vi "ConfigureDlg.vi"(8 "error in (no error)":errorcluster, 11 "PXI_MultiTrig in":refnum<class "PXI_MultiTrig.lvclass">) -> (0 "error out":errorcluster, 2 "Changed?":bool, 3 "PXI_MultiTrig out":refnum<class "PXI_MultiTrig.lvclass">)   [LabVIEW 2018, in "SyncPlugins.lvlib" / "PXI_MultiTrig.lvclass"]
uses:
  PXI_MultiTrig.lvclass
  C:/Program Files/National Instruments/LabVIEW 2018/user.lib/NIST/BaseClasses/BasePlugin_class/BasePlugin.lvclass
  Typedefs/clClocks.ctl
  Typedefs/clTrigger.ctl
  Typedefs/TimeRefType.ctl
  PXI_MultiTrig.lvclass/PXI_MultiTrig.ctl
  <userlib>/NIST/BaseClasses/BasePlugin_class/BasePlugin.lvclass/BasePlugin.ctl
  Accessors/Read RefClkHandle.vi
  Accessors/Read TimingHandle.vi
  Accessors/Read Clocks.vi
  Accessors/Read Triggers.vi
  Accessors/Read TimeRefType.vi
  Accessors/Read SyncWindowsClock.vi
  Accessors/Read RefClkSource.vi
  Accessors/Write RefClkHandle.vi
  Accessors/Write TimingHandle.vi
  Accessors/Write Clocks.vi
  Accessors/Write Triggers.vi
  <userlib>/NIST/BaseClasses/BasePlugin_class/Accessors/Read PluginIniFilePath.vi
  Accessors/Write TimeRefType.vi
  Accessors/Write SyncWindowsClock.vi
  Accessors/Write RefClkSource.vi
  <userlib>/NIST/BaseClasses/BasePlugin_class/Accessors/Write PluginIniFilePath.vi
  <vilib>/Utility/config.llb/NI_LVConfig.lvlib
panel:
  in  "btnSaveAs":bool
  in  "btnSave":bool
  in  "Tab Control":T1(tab)
  in  "TimingCard":string="PXI1Slot7"
  in  "TimeRefType":T2=enum."GPS"
  in  "SyncWinClk":bool caption="Synchronize Windows Clock"
  in  "RefClkSource":string="PXI_Trig0"
  in  "RefClkCard":string="PXI1Slot7"
  in  "Clocks":T3[](array[typedef])
  in  "Triggers":T4[](array[typedef]) {"Invert?" items=["Don't Invert Signal", "Invert Signal"]; "Edge" items=["Rising Edge", "Falling Edge"]}
  in  "btnCancel":bool
  # "Windows clock synchronization\nrequires LabVIEW to be running\nas Administrator"
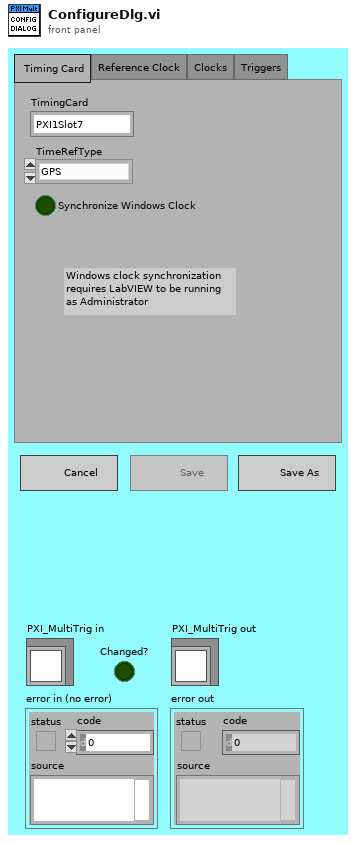
[diagram p1: front panel]
types:
  T1 = enum32{" Timing Card", "Reference Clock", "Clocks", "Triggers"}
  T2 = typedef "SyncPlugins.lvlib/PXI_MultiTrig.lvclass/TimeRefType.ctl" = enum16{"1588", "Free Running", "GPS", "IRIG", "PPS"}
  T3 = typedef "SyncPlugins.lvlib/PXI_MultiTrig.lvclass/clClocks.ctl" = cluster{"Name":string, "RefClk":string, "ClkTerminal":string, "Frequency":dbl, "DutyCycle":dbl, "ClkType":string, "Initiated":bool, "TrigTime":bool}
  T4 = typedef "SyncPlugins.lvlib/PXI_MultiTrig.lvclass/clTrigger.ctl" = cluster{"Name":string, "DestTerm":string, "SrcTerm":string, "SyncClk":string, "Edge":i32, "Invert?":i32, "Initiated":bool, "Type":string, "TrigTime":bool}
  T5 = enum8{"Enabled", "Disabled", "Disabled and Grayed Out"}
  T6 = enum32{"Invalid", "Default", "Floating", "Floating/Auto-Hide", "Modal"}
  T7 = typedef "NI_LVConfig.lvlib/Config Data RefNum.ctl" = refnum<k1>
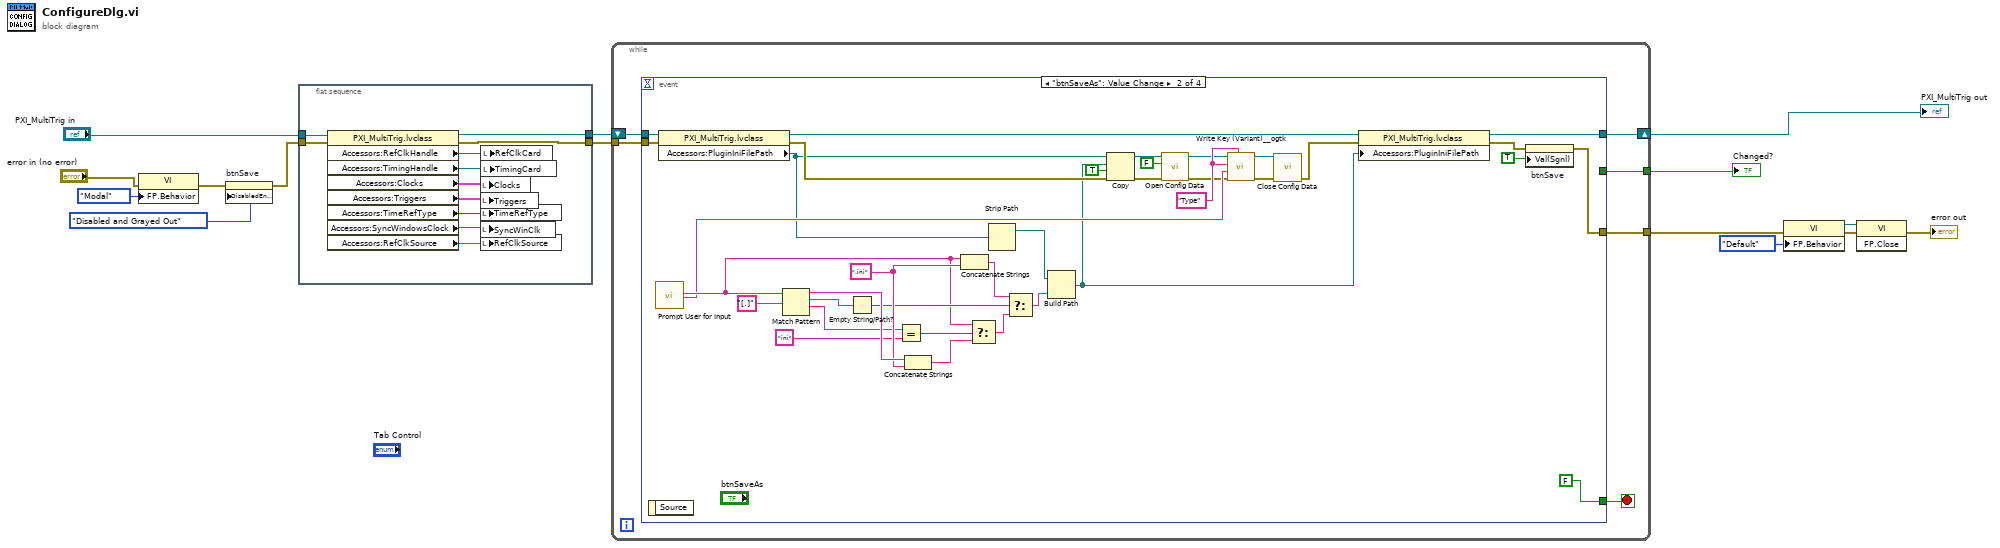
[diagram p0: block diagram]
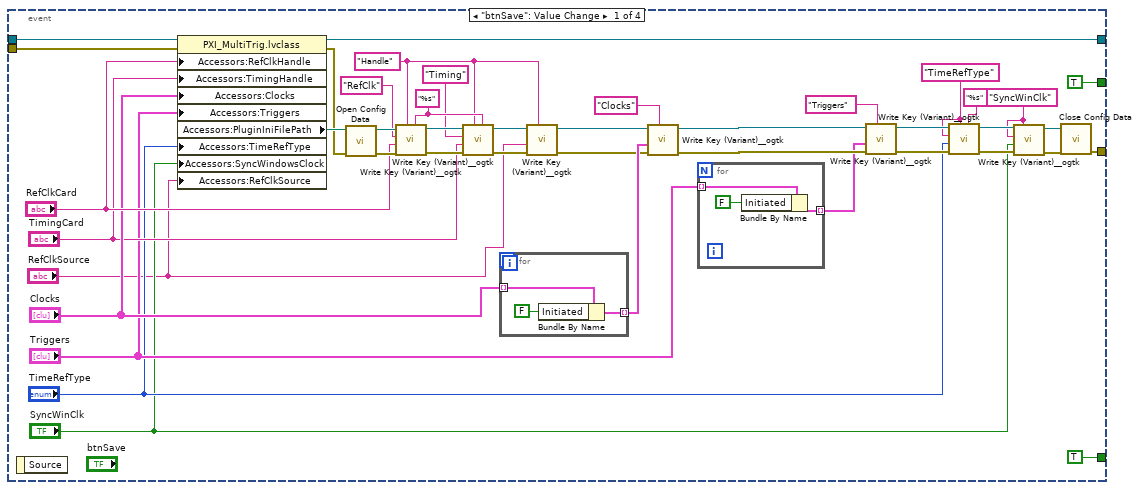
[diagram p2: hidden frame]
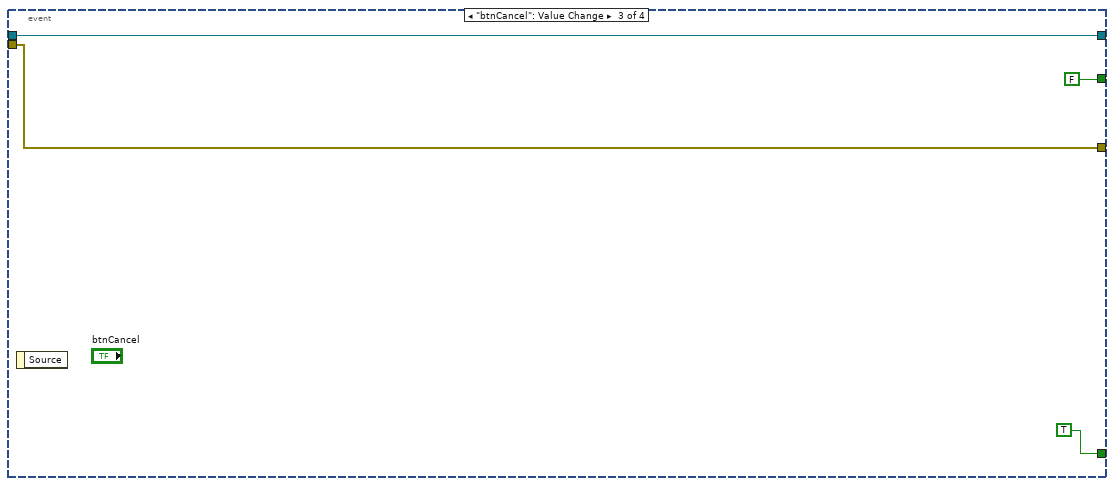
[diagram p3: hidden frame]
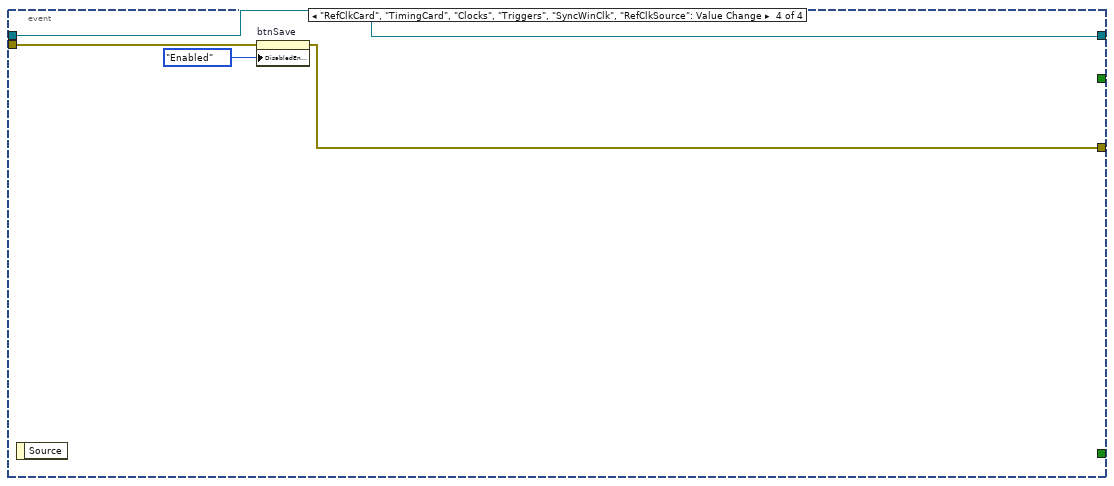
[diagram p4: hidden frame]
diagram:
  n1 = property class="VI"(error in="error in (no error)", "FP.Behavior"=T6."Modal" ("Front Panel Window:Behavior")) -> (error out=w3:errorcluster)  [unwired: 1 in, 1 out]
  n2 = property on="btnSave" class="Bool (strict)"(error in=w3, "DisabledEnum"=T5."Disabled and Grayed Out" ("Disabled")) -> (error out=w2:errorcluster)  [unwired: 1 in, 1 out]
  n3 = flat-sequence {
    tunnel: "PXI_MultiTrig in" -> [w26]
    tunnel: [w25] -> w14
    tunnel: w2 -> [w24]
    tunnel: [w16] -> w4
    frame #0 {
      n4 = property class="PXI_MultiTrig.lvclass"(reference=w26, error in=w24) -> (reference out=w25:refnum<class "PXI_MultiTrig.lvclass">, error out=w16:errorcluster, "Accessors:RefClkHandle"=w23:refnum<k15>, "Accessors:TimingHandle"=w22:refnum<k15>, "Accessors:Clocks"=w21:T3[], "Accessors:Triggers"=w20:T4[], "Accessors:TimeRefType"=w19:T2, "Accessors:SyncWindowsClock"=w18:bool, "Accessors:RefClkSource"=w17:string)
      n5 = local write "Clocks"(w21) -> ()
      n6 = local write "Triggers"(w20) -> ()
      n7 = local write "TimeRefType"(w19) -> ()
      n8 = local write "SyncWinClk"(w18) -> ()
      n9 = local write "RefClkSource"(w17) -> ()
      n10 = local write "RefClkCard"(w23) -> ()
      n11 = local write "TimingCard"(w22) -> ()
    }
  }
  n12 = while {
    tunnel: [w31] -> w8
    tunnel: [w30] -> w6
    shift-right: [w29] -> w5
    shift-left: w14 -> [w32]
    tunnel: w4 -> [w27]
    stop <- w28 stop-if-true
    n13 = event shown="[1] \"btnSaveAs\": Value Change" {
      selector: _ -> [_ _ _ _]
      dyn-events: _ -> [_ _ _ _]
      timeout: _ -> [_ _ _ _]
      tunnel: w32 -> [w74 w103 w119 w122]
      tunnel: w27 -> [w73 w102 w120 w124]
      tunnel: [w57 w96 w120 w121] -> w31
      tunnel: [TRUE _ FALSE _] -> w30
      tunnel: [w55 w97 w119 w122] -> w29
      tunnel: [TRUE FALSE TRUE _] -> w28
      event "btnSave": Value Change {
        w45 = "SyncWinClk" ("section")
        w51 = "TimeRefType" ("section")
        w34 = "Handle" ("section")
        w64 = "%s" ("float number format")
        n14 = event-data() -> ()  [unwired: 1 in, 1 out]
        n15 = property class="PXI_MultiTrig.lvclass"(reference=w74, error in=w73, "Accessors:RefClkHandle"="RefClkCard", "Accessors:TimingHandle"="TimingCard", "Accessors:Clocks"="Clocks", "Accessors:Triggers"="Triggers", "Accessors:TimeRefType"="TimeRefType", "Accessors:SyncWindowsClock"="SyncWinClk", "Accessors:RefClkSource"="RefClkSource") -> (reference out=w55:refnum<class "PXI_MultiTrig.lvclass">, error out=w71:errorcluster, "Accessors:PluginIniFilePath"=w72:path)
        n16 = call <vilib>:"Open Config Data.vi"("error in (no error)"=w71, "configuration file path"=w72) -> ("error out"=w70:errorcluster, "refnum"=w69:T7)  [unwired: 7 in, 1 out]
        n17 = call <userlib>:"Write Key (Variant)__ogtk.vi"("float number format"=w64, "section"=w34, "error in (no error)"=w70, "key-value"="RefClkCard", "key (optional)"="RefClk", "refnum"=w69) -> ("error out"=w66:errorcluster, "refnum out"=w65:T7)  [unwired: 4 in]
        n18 = call <userlib>:"Write Key (Variant)__ogtk.vi"("float number format"=w64, "section"=w34, "error in (no error)"=w66, "key-value"="TimingCard", "key (optional)"="Timing", "refnum"=w65) -> ("error out"=w38:errorcluster, "refnum out"=w37:T7)  [unwired: 4 in]
        n19 = for {
          tunnel: "Clocks" -> [w80] mode=indexing
          tunnel: [w79] -> w43 mode=indexing
          n20 = Bundle By Name(cluster=w80, "Initiated"=FALSE) -> (w79:T3)
        }
        n21 = call <userlib>:"Write Key (Variant)__ogtk.vi"("section"=w34, "error in (no error)"=w38, "key-value"="RefClkSource", "refnum"=w37) -> ("error out"=w35:errorcluster, "refnum out"=w36:T7)  [unwired: 6 in]
        n22 = call <userlib>:"Write Key (Variant)__ogtk.vi"("section"="Clocks", "error in (no error)"=w35, "key-value"=w43, "refnum"=w36) -> ("error out"=w59:errorcluster, "refnum out"=w58:T7)  [unwired: 6 in]
        n23 = for {
          tunnel: "Triggers" -> [w77] mode=indexing
          tunnel: [w76] -> w41 mode=indexing
          n24 = Bundle By Name(cluster=w77, "Initiated"=FALSE) -> (w76:T4)
        }
        n25 = call <userlib>:"Write Key (Variant)__ogtk.vi"("section"="Triggers", "error in (no error)"=w59, "key-value"=w41, "refnum"=w58) -> ("error out"=w54:errorcluster, "refnum out"=w53:T7)  [unwired: 6 in]
        n26 = call <userlib>:"Write Key (Variant)__ogtk.vi"("float number format"="%s", "section"=w51, "error in (no error)"=w54, "key-value"="TimeRefType", "key (optional)"=w51, "refnum"=w53) -> ("error out"=w49:errorcluster, "refnum out"=w48:T7)  [unwired: 4 in]
        n27 = call <userlib>:"Write Key (Variant)__ogtk.vi"("section"=w45, "error in (no error)"=w49, "key-value"="SyncWinClk", "key (optional)"=w45, "refnum"=w48) -> ("error out"=w46:errorcluster, "refnum out"=w47:T7)  [unwired: 5 in]
        n28 = call <vilib>:"Close Config Data.vi"("error in (no error)"=w46, "refnum"=w47) -> ("error out"=w57:errorcluster)  [unwired: 8 in, 1 out]
      }
      event "btnSaveAs": Value Change {
        w91 = "Type" ("key (optional)")
        w114 = ".ini" ("string")
        n29 = event-data() -> ()  [unwired: 1 in, 1 out]
        n30 = call "Prompt User for Input"() -> ("File Name"=w105:string, "PluginType"=w90:string)  [unwired: 16 in, 2 out]
        n31 = property class="PXI_MultiTrig.lvclass"(reference=w103, error in=w102) -> (reference out=w99:refnum<class "PXI_MultiTrig.lvclass">, error out=w87:errorcluster, "Accessors:PluginIniFilePath"=w85:path)
        n32 = Match Pattern(string=w105, regular expression="[.]" ("string")) -> (before substring=w115:string, match substring=w111:string, after substring=w112:string)  [unwired: 1 in, 1 out]
        n33 = Empty String/Path?(string/path=w111) -> (empty?=w106:bool)
        n34 = Equal?(x=w112, y="ini" ("string")) -> (x = y?=w108:bool)
        n35 = Concatenate Strings(w115, w114) -> (w116:string)
        n36 = Concatenate Strings(w105, w114) -> (w107:string)
        n37 = Select(t=w105, s=w108, f=w116) -> (s? t:f=w109:string)
        n38 = Strip Path(path=w85) -> (stripped path=w101:path)  [unwired: 1 out]
        n39 = Select(t=w107, s=w106, f=w109) -> (s? t:f=w104:string)
        n40 = Build Path(base path=w101, name or relative path=w104) -> (appended path=w84:path)
        n41 = Copy(8:w87, 9:TRUE ("overwrite (F)"), 10:w84, 11:w85) -> (0:w86:errorcluster, 3:w83:path)  [unwired: 1 in, 1 out]
        n42 = call <vilib>:"Open Config Data.vi"("error in (no error)"=w86, "create file if necessary (T)"=FALSE, "configuration file path"=w83) -> ("error out"=w88:errorcluster, "refnum"=w89:T7)  [unwired: 6 in, 1 out]
        n43 = call <userlib>:"Write Key (Variant)__ogtk.vi"("section"=w91, "error in (no error)"=w88, "key-value"=w90, "key (optional)"=w91, "refnum"=w89) -> ("error out"=w94:errorcluster, "refnum out"=w93:T7)  [unwired: 5 in]
        n44 = call <vilib>:"Close Config Data.vi"("error in (no error)"=w94, "refnum"=w93) -> ("error out"=w92:errorcluster)  [unwired: 8 in, 1 out]
        n45 = property class="PXI_MultiTrig.lvclass"(reference=w99, error in=w92, "Accessors:PluginIniFilePath"=w84) -> (reference out=w97:refnum<class "PXI_MultiTrig.lvclass">, error out=w98:errorcluster)
        n46 = property on="btnSave" class="Bool (strict)"(error in=w98, "Val(Sgnl)"=TRUE) -> (error out=w96:errorcluster)  [unwired: 1 in, 1 out]
      }
      event "btnCancel": Value Change {
        n47 = event-data() -> ()  [unwired: 1 in, 1 out]
      }
      event "RefClkCard", "TimingCard", "Clocks", "Triggers", "SyncWinClk", "RefClkSource": Value Change {
        n48 = event-data() -> ()  [unwired: 1 in, 1 out]
        n49 = property on="btnSave" class="Bool (strict)"(error in=w124, "DisabledEnum"=T5."Enabled" ("Disabled")) -> (error out=w121:errorcluster)  [unwired: 1 in, 1 out]
      }
    }
  }
  "PXI_MultiTrig out" <- w5
  "Changed?" <- w6
  n50 = property class="VI"(error in=w8, "FP.Behavior"=T6."Default" ("Front Panel Window:Behavior")) -> (reference out=w9:refnum<vi>, error out=w10:errorcluster)  [unwired: 1 in]
  n51 = invoke class="VI" method="FP.Close"(reference=w9, error in=w10) -> (error out=→"error out":errorcluster)  [unwired: 1 in, 2 out]
